vi "End of process.vi"(0 "Arduino Resource In":T1={"VISA resource"="", "Board Type"=enum."Uno", "Connection Type"=enum."USB / Serial", "Bytes Per Packet (15)"=15}, 5 "Error In":errorcluster) -> (14 "Arduino Resource Out":T1={"VISA resource"="", "Board Type"=enum."Uno", "Connection Type"=enum."USB / Serial", "Bytes Per Packet (15)"=15}, 19 "Error Out":errorcluster)   [LabVIEW 2016]
uses:
  <vilib>/LabVIEW Interface for Arduino/Type Defs/Arduino Resource.ctl
  <vilib>/LabVIEW Interface for Arduino/Type Defs/Board Type.ctl
  <vilib>/LabVIEW Interface for Arduino/LabVIEW Interface for Arduino.lvlib
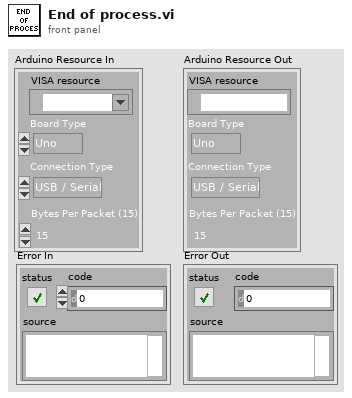
[diagram p1: front panel]
types:
  T1 = typedef "LabVIEW Interface for Arduino.lvlib/Arduino Resource.ctl" = cluster{"VISA resource":refnum<visa-resource-name>, "Board Type":T2, "Connection Type":enum8{"USB / Serial"}, "Bytes Per Packet (15)":u8}
  T2 = typedef "LabVIEW Interface for Arduino.lvlib/Board Type.ctl" = enum16{"Uno", "Dimuelanove w/Atmega 328", "Mega 2560"}
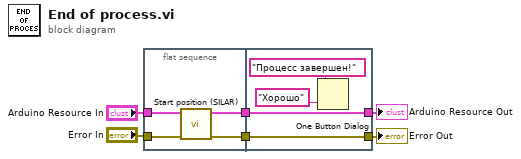
[diagram p0: block diagram]
diagram:
  n1 = flat-sequence {
    tunnel: "Arduino Resource In" -> [w10]
    tunnel: [w9] -> w6
    tunnel: [w8] -> w5
    tunnel: "Error In" -> [w7]
    tunnel: [w13] -> w1
    tunnel: [w14] -> w2
    tunnel: w6 -> [w14]
    tunnel: w5 -> [w13]
    frame #0 {
      n2 = call "Start position (SILAR).vi"("Error In"=w7, "Arduino Resource In"=w10) -> ("Error Out"=w8:errorcluster, "Arduino Resource Out"=w9:T1)  [unwired: 8 in]
    }
    frame #1 {
      n3 = One Button Dialog(message="Процесс завершен!", button name ("OK")="Хорошо") -> ()  [unwired: 1 out]
    }
  }
  "Arduino Resource Out" <- w2
  "Error Out" <- w1
